vi "Enter WebDAV Credentials.vi"(8 "error in (no error)":errorcluster, 10 "IP Address":string, 11 "host uri prefix":string) -> (0 "error out":errorcluster, 1 "Password Output":string, 2 "Username Output":string, 3 "WebDAV session handle out":T1)   [LabVIEW 2014]
doc: "Prompts the user to input a username and password for WebDAV connection"
uses:
  <vilib>/WebDAVClient/Advanced/SessionHandle.ctl
  <vilib>/WebDAVClient/NI_WebDAV.lvlib
panel:
  out "Prompt":string caption="Current action:"
  in  "Cancel":bool
  in  "Ok":bool
  in  "Password":string
  in  "Username":string
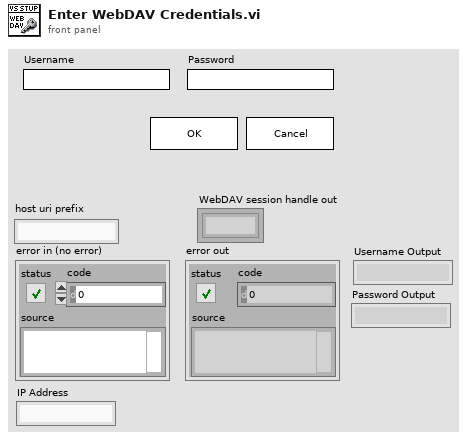
[diagram p1: front panel]
types:
  T1 = typedef "NI_WebDAV.lvlib/SessionHandle.ctl" = refnum<k1>
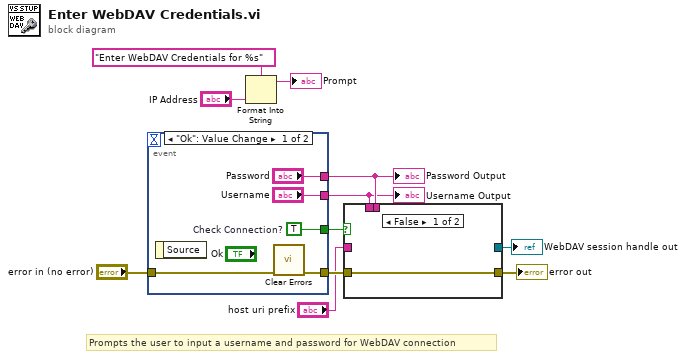
[diagram p0: block diagram]
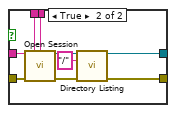
[diagram p2: hidden frame]
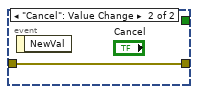
[diagram p3: hidden frame]
diagram:
  # "Prompts the user to input a username and password for WebDAV connection"
  n1 = event shown="[0] \"Ok\": Value Change" {
    selector: _ -> [_ _]
    dyn-events: _ -> [_ _]
    timeout: _ -> [_ _]
    tunnel: "error in (no error)" -> [w15 w17]
    tunnel: [w16 w17] -> w10
    tunnel: [w14 _] -> w5
    tunnel: ["Username" _] -> w8
    tunnel: ["Password" _] -> w9
    event "Ok": Value Change {
      w14 = TRUE  # Check Connection?
      n2 = event-data() -> ()  [unwired: 1 in, 1 out]
      n3 = call <vilib>:"Clear Errors.vi"("error in (no error)"=w15) -> ("error out"=w16:errorcluster)  [unwired: 5 in, 1 out]
    }
    event "Cancel": Value Change {
      n4 = event-data() -> ()  [unwired: 1 in, 1 out]
    }
  }
  "Username Output" <- w8
  "Password Output" <- w9
  n5 = Format Into String(format string="Enter WebDAV Credentials for %s" ("Prompt"), "IP Address") -> (resulting string=→"Prompt":string)  [unwired: 2 in, 1 out]
  n6 = case shown="False" w5 {
    tunnel: w10 -> [w18 w27]
    tunnel: w9 -> [_ w26]
    tunnel: w8 -> [_ w25]
    tunnel: "host uri prefix" -> [_ w24]
    tunnel: [w18 w20] -> w6
    tunnel: [_ w19] -> w1
    frame False {
    }
    frame True {
      n7 = call <vilib>:"Open Session.vi"("host uri prefix"=w24, "username"=w25, "password"=w26, "error in (no error)"=w27) -> ("session handle out"=w23:T1, "error out"=w22:errorcluster)  [unwired: 10 in]
      n8 = call <vilib>:"Directory Listing.vi"("session handle"=w23, "relative uri"="/", "error in (no error)"=w22) -> ("session handle out"=w19:T1, "error out"=w20:errorcluster)  [unwired: 9 in, 2 out]
    }
  }
  "error out" <- w6
  "WebDAV session handle out" <- w1
